vi "Localisation.vi"(8 "x2":dbl caption="Distance de l'objet par rapport au centre de l'écran de la caméra 2", 10 "x1":dbl caption="Distance de l'objet par rapport au centre de l'écran de la caméra 1", 11 "b":dbl caption="Moitié de l'écran à horizontale pour les 2 caméras") -> (1 "d":string caption="Distance de l'objet par rapport à la tourelle en mètre")   [LabVIEW 2013]
panel:
  # "Algorithme de calcul de distance par stéréoscopie"
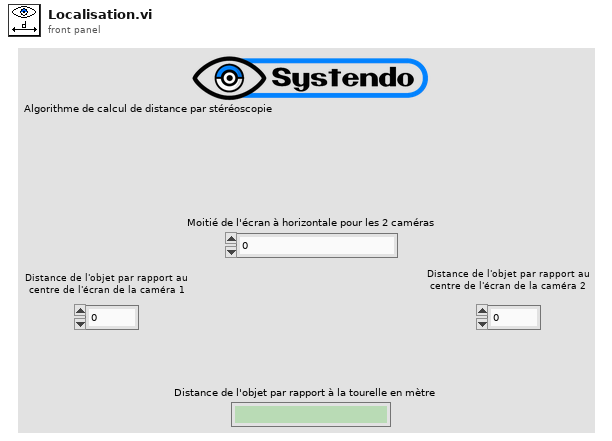
[diagram p1: front panel]
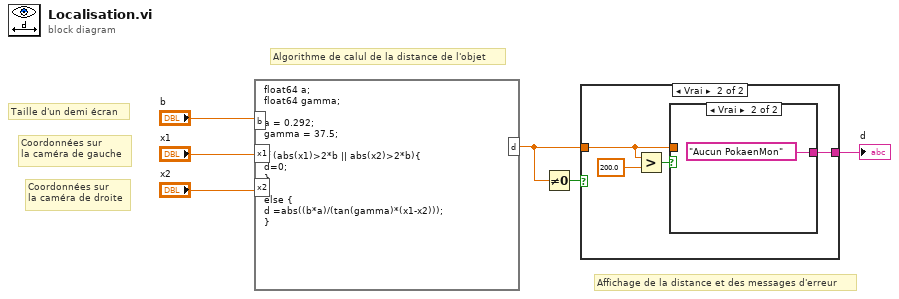
[diagram p0: block diagram]
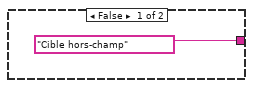
[diagram p2: hidden frame]
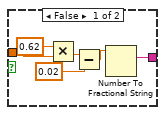
[diagram p3: hidden frame]
diagram:
  # "Affichage de la distance et des messages d'erreur"
  # "Coordonnées sur\nla caméra de droite"
  # "Coordonnées sur\nla caméra de gauche"
  # "Taille d'un demi écran"
  # "Algorithme de calul de la distance de l'objet"
  n1 = formula code="float64 a;\nfloat64 gamma;\n\na = 0.292;\ngamma = 37.5;\n\nif (abs(x1)>2*b || abs(x2)>2*b){\nd=0;\n}\n\nelse {\nd =abs((b*a)/(tan(gamma)*(x1-x2)));\n}"("b"="b", "x1"="x1", "x2"="x2") -> ("d"=w2:dbl)
  n2 = Not Equal To 0?(x=w2) -> (x != 0?=w3:bool)
  n3 = case shown="Vrai" w3 {
    tunnel: w2 -> [_ w9]
    tunnel: ["Cible hors-champ" w11] -> w1
    frame False {
    }
    frame True {
      n4 = Greater?(x=w9, y=200.0) -> (0:w10:bool)
      n5 = case shown="Vrai" w10 {
        tunnel: [w12 "Aucun PokaenMon"] -> w11
        tunnel: w9 -> [w13 _]
        frame False {
          n6 = Multiply(x=0.62, y=w13) -> (x*y=w16:dbl)
          n7 = Subtract(x=w16, y=0.02) -> (x-y=w15:dbl)
          n8 = Number To Fractional String(number=w15) -> (F-format string=w12:string)  [unwired: 3 in]
        }
        frame True {
        }
      }
    }
  }
  "d" <- w1
